vi "firmware version.vi"() -> (0 "target firmware version":dbl=4.0)   [LabVIEW 2017]
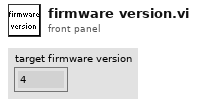
[diagram p1: front panel]
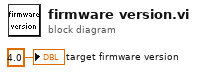
[diagram p0: block diagram]
diagram:
  "target firmware version" <- 4.0
